vi "saveCalFile.vi"(7 "LWSR":refnum<class "Web Request.lvclass">, 10 "file_name":string) -> ()   [LabVIEW 2014]
uses:
  <vilib>/wsapi/Web Request.lvclass
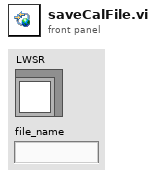
[diagram p1: front panel]
types:
  T1 = enum16{"open", "replace", "create", "open or create", "replace or create", "replace or create with confirmation"}
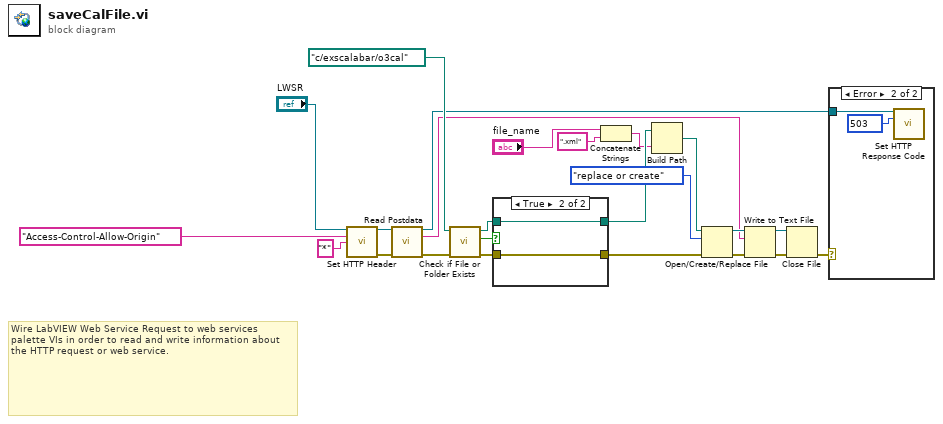
[diagram p0: block diagram]
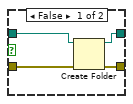
[diagram p2: hidden frame]
diagram:
  # "Wire LabVIEW Web Service Request to web services palette VIs in order to read and write information about the HTTP request or web service."
  n1 = call <vilib>:"Set HTTP Header.vi"("LabVIEW Web Service Request"="LWSR", "header"="Access-Control-Allow-Origin", "header value"="*") -> ("LabVIEW Web Service Request out"=w2:refnum<class "Web Request.lvclass">, "error out"=w1:errorcluster)  [unwired: 11 in]
  n2 = call <vilib>:"Read Postdata.vi"("LabVIEW Web Service Request"=w2, "error in (no error)"=w1) -> ("LabVIEW Web Service Request out"=w8:refnum<class "Web Request.lvclass">, "postdata"=w6:string, "error out"=w7:errorcluster)  [unwired: 11 in]
  n3 = call <vilib>:"Check if File or Folder Exists.vi"("error in (no error)"=w7, "path"=path "c:/exscalabar/o3cal" ("file path (use dialog)")) -> ("error out"=w14:errorcluster, "file or folder exists?"=w16:bool, "dup path"=w15:path)  [unwired: 7 in]
  n4 = case shown="True" w16 {
    tunnel: w15 -> [w28 w30]
    tunnel: w14 -> [w27 w29]
    tunnel: [w26 w30] -> w13
    tunnel: [w25 w29] -> w12
    frame False {
      n5 = Create Folder(path (use dialog)=w28, error in=w27) -> (created path=w26:path, error out=w25:errorcluster)  [unwired: 1 in, 1 out]
    }
    frame True {
    }
  }
  n6 = Concatenate Strings("file_name", ".xml" ("string")) -> (w9:string)
  n7 = Build Path(base path=w13, name or relative path=w9) -> (appended path=w23:path)
  n8 = Open/Create/Replace File(file path (use dialog)=w23, error in=w12, operation (0:open)=T1."replace or create") -> (refnum out=w22:refnum<file>, error out=w21:errorcluster)  [unwired: 3 in, 1 out]
  n9 = Write to Text File(file (use dialog)=w22, text=w6, error in=w21) -> (refnum out=w20:refnum<file>, error out=w19:errorcluster)  [unwired: 1 in, 1 out]
  n10 = Close File(refnum=w20, error in=w19) -> (error out=w18:errorcluster)  [unwired: 1 out]
  n11 = case shown="Error" w18 {
    tunnel: w8 -> [_ w31]
    frame No Error {
    }
    frame Error {
      w32 = 503 items=["100"=100, "101"=101, "200"=200, "201"=201, "202"=202, "203"=203, "204"=204, "205"=205, "206"=206, "300"=300, "301"=301, "302"=302, "303"=303, "304"=304, "305"=305, "306"=306, "307"=307, "400"=400, "401"=401, "402"=402, "403"=403, "404"=404, "405"=405, "406"=406, "407"=407, "408"=408, "409"=409, "410"=410, "411"=411, "412"=412, "413"=413, "414"=414, "415"=415, "416"=416, "417"=417, "500"=500, "501"=501, "502"=502, "503"=503, "504"=504, "505"=505] ("response code (200)")
      n12 = call <vilib>:"Set HTTP Response Code.vi"("LabVIEW Web Service Request"=w31, "response code (200)"=w32) -> ()  [unwired: 12 in, 2 out]
    }
  }
